vi "Write to TDMS.vi"(8 "error in (no error)":errorcluster, 10 "TDMS File Ref":refnum<k34>, 11 "Logging Data Interface in":refnum<class "Logging Data Interface.lvclass">) -> (0 "error out":errorcluster)   [LabVIEW 2024, in "Logging Data Interface.lvlib" / "Logging Data Interface.lvclass"]
uses:
  Logging Data Interface.lvclass
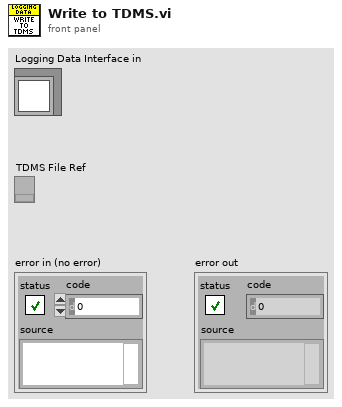
[diagram p1: front panel]
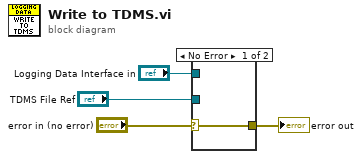
[diagram p0: block diagram]
diagram:
  n1 = case shown="No Error" "error in (no error)" {
    selector: "error in (no error)" -> [w5 w6]
    tunnel: [w5 w6] -> w3
    tunnel: "Logging Data Interface in" -> [_ _]
    tunnel: "TDMS File Ref" -> [_ _]
    frame No Error {
    }
    frame Error {
    }
  }
  "error out" <- w3
